vi "niSwitch Close gRPC Session.vi"(8 "error in":errorcluster, 11 "session factory in":refnum<class "Session Factory.lvclass">) -> (0 "error out":errorcluster)   [LabVIEW 2021, in "Session Management niSwitch.lvlib" / "Session Factory.lvclass"]
doc: "Closes the session specified in <b>session factory in</b> and deallocates the resources that NI-Switch reserved."
uses:
  Session Factory.lvclass
  Session Factory.lvclass/Session Factory.ctl
  NI Switch Client/NI Switch Client.lvlib
  NI Switch Client/RPC Messages/nidevice_grpc_Session_session/nidevice_grpc_Session_session.lvclass
  NI Switch Client/RPC Messages/nidevice_grpc_Session.ctl
  NI Switch Client/RPC Messages/niswitch_grpc_CloseRequest.ctl
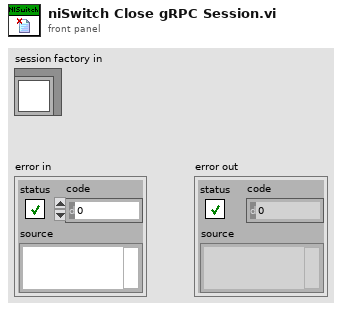
[diagram p1: front panel]
types:
  T1 = typedef "NI Switch Client.lvlib/niswitch_grpc_CloseRequest.ctl" = cluster{"vi":T2}
  T2 = typedef "NI Switch Client.lvlib/nidevice_grpc_Session.ctl" = cluster{"nidevice_grpc_Session_session":refnum<class "nidevice_grpc_Session_session.lvclass">}
  T3 = typedef "grpc-lvsupport-release.lvlib/grpcId.ctl" = u64
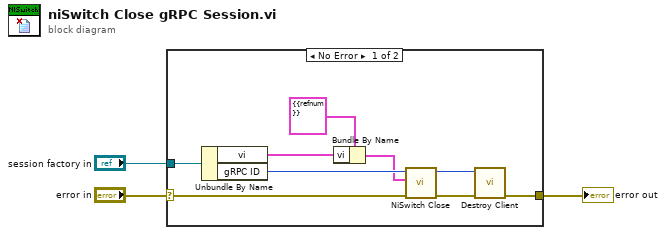
[diagram p0: block diagram]
diagram:
  n1 = case shown="No Error" "error in" {
    selector: "error in" -> [w8 w13]
    tunnel: [w6 w13] -> w3
    tunnel: "session factory in" -> [w4 _]
    frame No Error {
      n2 = Unbundle By Name(w4) -> ("vi"=w11:T2, "gRPC ID"=w12:T3)
      n3 = Bundle By Name(cluster=T1 {"vi"={"nidevice_grpc_Session_session"=refnum}} ("Request Data"), "vi"=w11) -> (w9:T1)
      n4 = call "NiSwitch Close.vi"("error in"=w8, "Request Data"=w9, "gRPC ID"=w12) -> ("error out"=w7:errorcluster, "gRPC ID out"=w5:T3)  [unwired: 6 in, 1 out]
      n5 = call "Destroy Client.vi"("error in"=w7, "gRPC ID"=w5) -> ("error out"=w6:errorcluster)  [unwired: 9 in]
    }
    frame Error {
    }
  }
  "error out" <- w3
